vi "Master State Control.vi"(2 "Elevator_State":string) -> (0 "Elevator_State_Out":string, 1 "Target_Vacuum_Pump_Power":dbl)   [LabVIEW 2018]
uses:
  RefNumsDriverStation.vi
  Sensor Readings.vi
  Robot States.vi
panel:
  out "Target_Elevator_Position":dbl
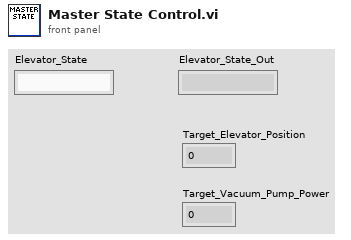
[diagram p1: front panel]
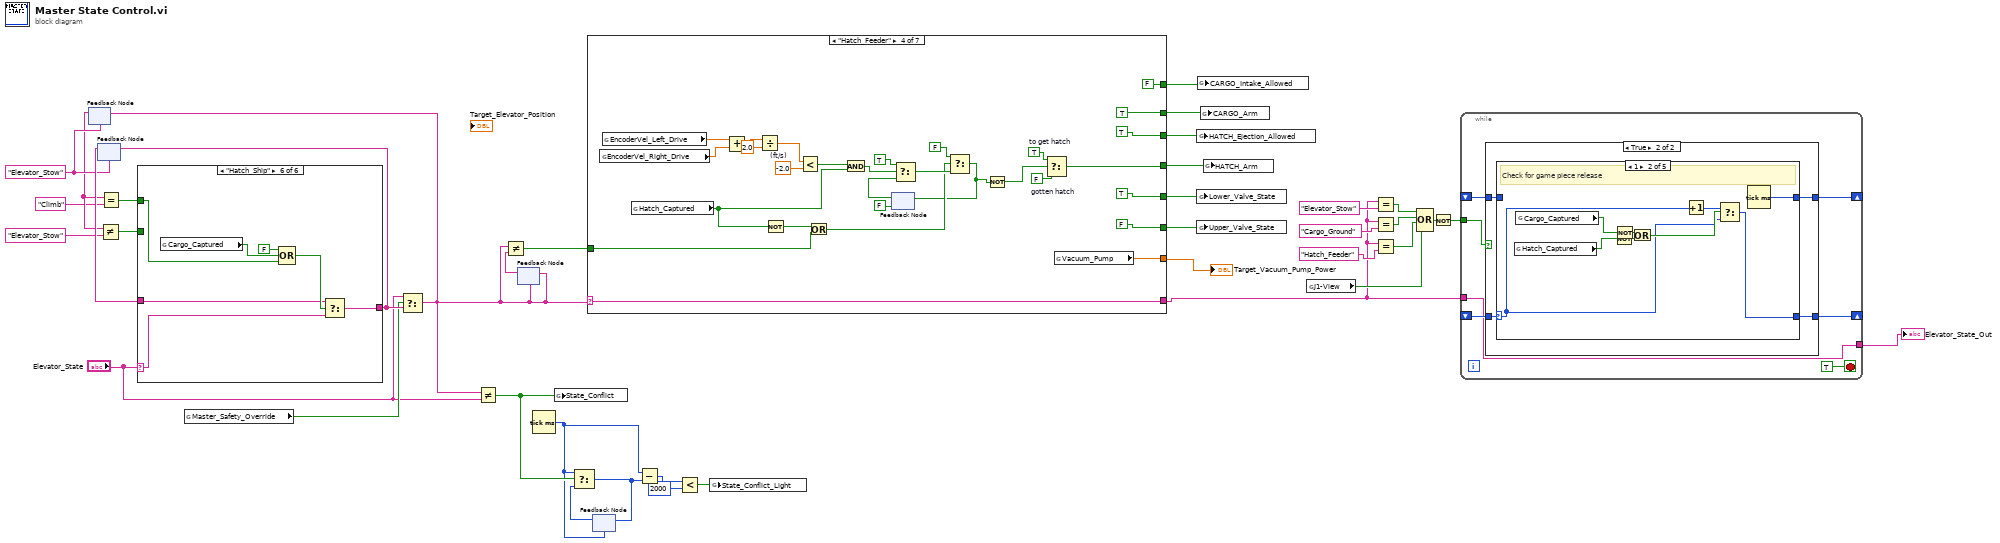
[diagram p0: block diagram]
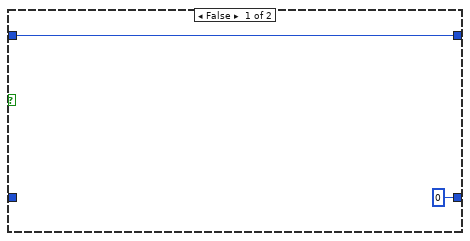
[diagram p2: hidden frame]
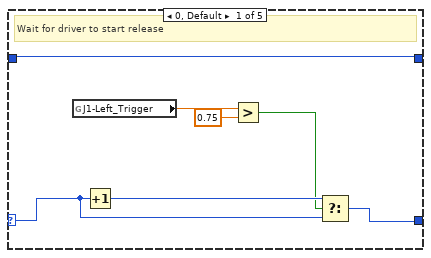
[diagram p3: hidden frame]
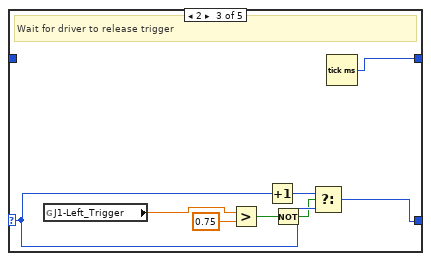
[diagram p4: hidden frame]
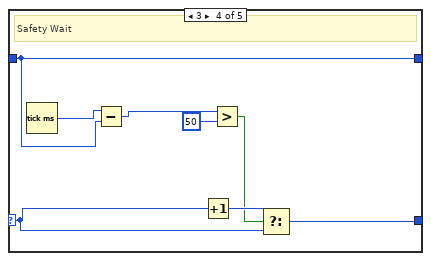
[diagram p5: hidden frame]
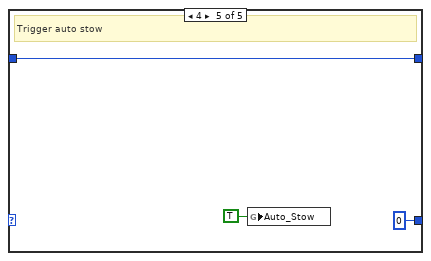
[diagram p6: hidden frame]
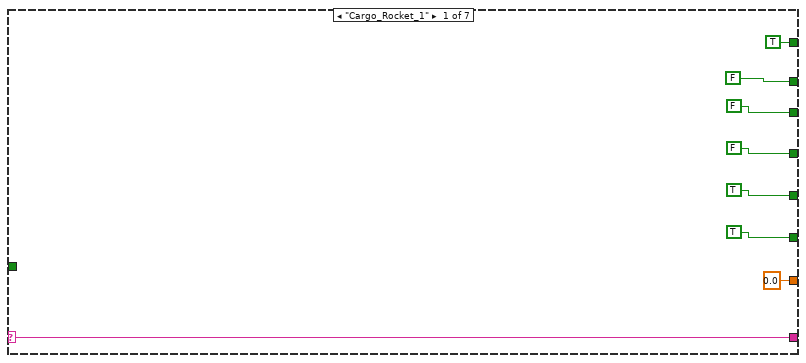
[diagram p7: hidden frame]
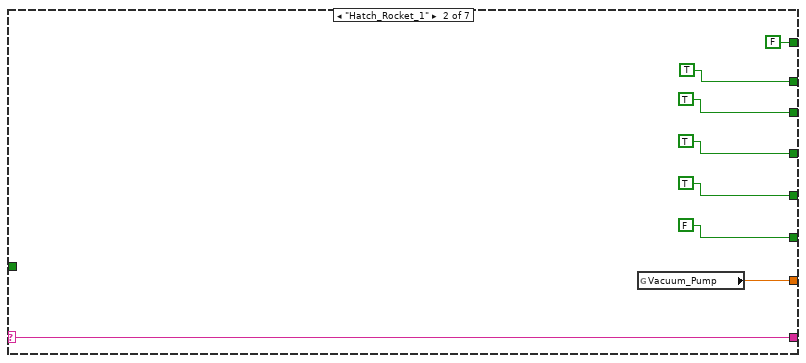
[diagram p8: hidden frame]
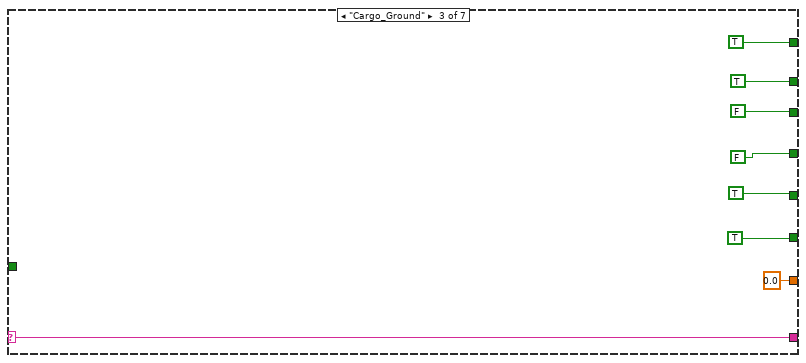
[diagram p9: hidden frame]
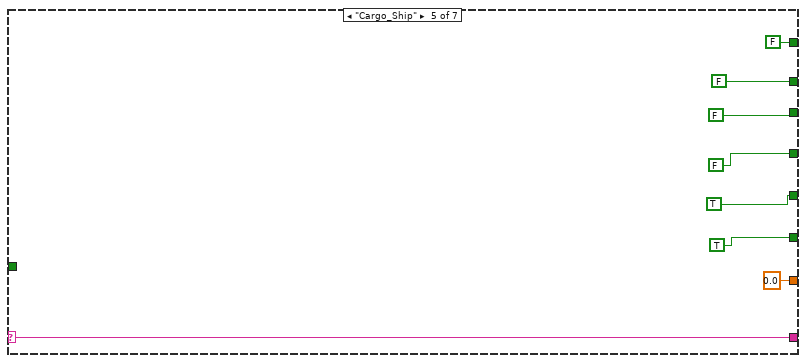
[diagram p10: hidden frame]
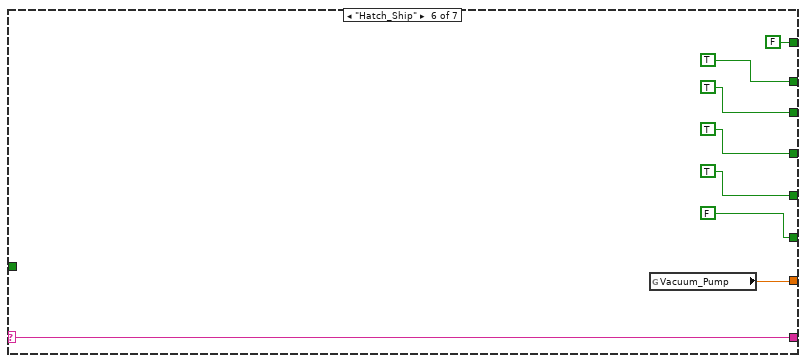
[diagram p11: hidden frame]
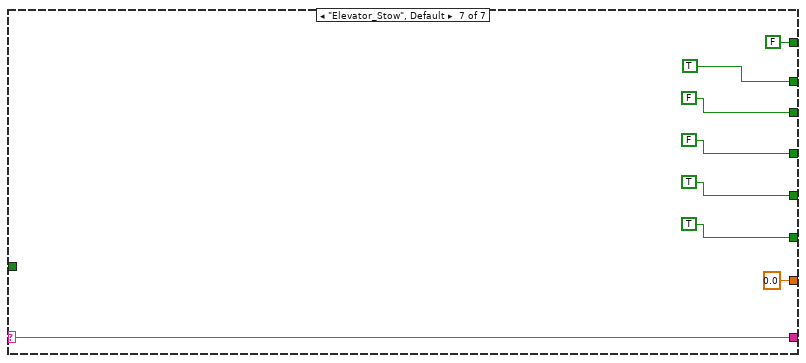
[diagram p12: hidden frame]
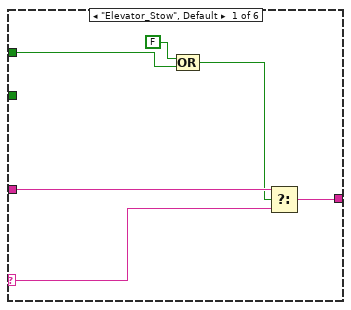
[diagram p13: hidden frame]
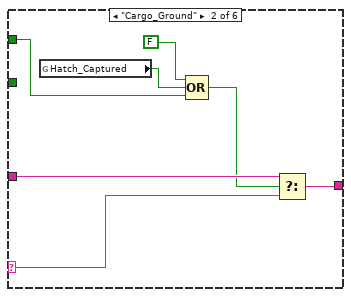
[diagram p14: hidden frame]
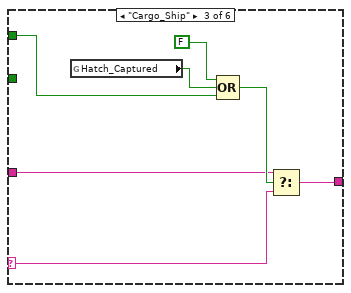
[diagram p15: hidden frame]
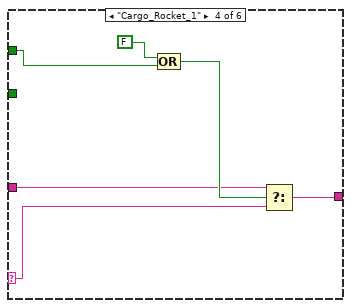
[diagram p16: hidden frame]
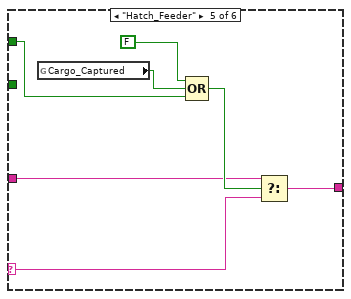
[diagram p17: hidden frame]
diagram:
  w36 = "Elevator_Stow" ("Elevator_State")
  n1 = feedback #1(w36) -> (w34:string)
  n2 = feedback #2(w36) -> (w38:string)
  n3 = Not Equal?(x=w34, y="Elevator_Stow") -> (x != y?=w32:bool)
  n4 = Equal?(x=w34, y="Climb") -> (x = y?=w31:bool)
  n5 = case shown="\"Hatch_Ship\"" "Elevator_State" {
    selector: "Elevator_State" -> [w39 w47 w54 w60 w66 w73]
    tunnel: [w44 w48 w55 w59 w65 w75] -> w37
    tunnel: w38 -> [w43 w46 w52 w61 w67 w72]
    tunnel: w32 -> [_ _ _ _ _ _]
    tunnel: w31 -> [w42 w51 w56 w64 w71 w78]
    frame "Elevator_Stow", Default {
      n6 = Compound Arithmetic op=OR(FALSE ("value"), w42) -> (w40:bool)
      n7 = Select(t=w43, s=w40, f=w39) -> (s? t:f=w44:string)
    }
    frame "Cargo_Ground" {
      n8 = global read "Sensor Readings.vi" "Hatch_Captured"() -> (w50:bool)
      n9 = Compound Arithmetic op=OR(FALSE ("value"), w50, w51) -> (w45:bool)
      n10 = Select(t=w46, s=w45, f=w47) -> (s? t:f=w48:string)
    }
    frame "Cargo_Ship" {
      n11 = global read "Sensor Readings.vi" "Hatch_Captured"() -> (w58:bool)
      n12 = Compound Arithmetic op=OR(FALSE ("value"), w58, w56) -> (w53:bool)
      n13 = Select(t=w52, s=w53, f=w54) -> (s? t:f=w55:string)
    }
    frame "Cargo_Rocket_1" {
      n14 = Compound Arithmetic op=OR(FALSE ("value"), w64) -> (w62:bool)
      n15 = Select(t=w61, s=w62, f=w60) -> (s? t:f=w59:string)
    }
    frame "Hatch_Feeder" {
      n16 = global read "Sensor Readings.vi" "Cargo_Captured"() -> (w70:bool)
      n17 = Compound Arithmetic op=OR(FALSE ("value"), w70, w71) -> (w68:bool)
      n18 = Select(t=w67, s=w68, f=w66) -> (s? t:f=w65:string)
    }
    frame "Hatch_Ship" {
      n19 = global read "Sensor Readings.vi" "Cargo_Captured"() -> (w77:bool)
      n20 = Compound Arithmetic op=OR(FALSE ("value"), w77, w78) -> (w74:bool)
      n21 = Select(t=w72, s=w74, f=w73) -> (s? t:f=w75:string)
    }
  }
  n22 = feedback-in #2(w37) -> ()
  n23 = global read "RefNumsDriverStation.vi" "Master_Safety_Override"() -> (w12:bool)
  n24 = Select(t="Elevator_State", s=w12, f=w37) -> (s? t:f=w1:string)
  n25 = feedback-in #1(w1) -> ()
  n26 = Not Equal?(x=w1, y="Elevator_State") -> (x != y?=w10:bool)
  n27 = feedback-in #3(w1) -> ()
  n28 = feedback #3(w1) -> (w3:string)
  n29 = Not Equal?(x=w1, y=w3) -> (x != y?=w2:bool)
  n30 = Tick Count (ms)() -> (millisecond timer value=w5:u32)
  n31 = global write "Robot States.vi" "State_Conflict"(w10) -> ()
  n32 = case shown="\"Hatch_Feeder\"" w1 {
    selector: w1 -> [w79 w94 w102 w131 w139 w147 w155]
    tunnel: [w79 w94 w102 w131 w139 w147 w155] -> w13
    tunnel: [0.0 ("Vacuum_Pump") w93 0.0 ("Vacuum_Pump") w130 0.0 ("Vacuum_Pump") w146 0.0 ("Vacuum_Pump")] -> w30
    tunnel: [FALSE TRUE FALSE TRUE FALSE TRUE FALSE] -> w29
    tunnel: [FALSE TRUE FALSE w103 FALSE TRUE FALSE] -> w28
    tunnel: [TRUE TRUE TRUE TRUE TRUE TRUE TRUE] -> w27
    tunnel: [TRUE FALSE TRUE FALSE TRUE FALSE TRUE] -> w26
    tunnel: [FALSE ("CARGO_Arm") TRUE ("CARGO_Arm") TRUE ("CARGO_Arm") TRUE ("CARGO_Arm") FALSE ("CARGO_Arm") TRUE ("CARGO_Arm") TRUE ("CARGO_Arm")] -> w25
    tunnel: [TRUE ("CARGO_Intake_Allowed") FALSE ("CARGO_Intake_Allowed") TRUE ("CARGO_Intake_Allowed") FALSE ("CARGO_Intake_Allowed") FALSE ("CARGO_Intake_Allowed") FALSE ("CARGO_Intake_Allowed") FALSE ("CARGO_Intake_Allowed")] -> w24
    tunnel: w2 -> [_ _ _ w111 _ _ _]
    frame "Cargo_Rocket_1" {
    }
    frame "Hatch_Rocket_1" {
      n33 = global read "RefNumsDriverStation.vi" "Vacuum_Pump"() -> (w93:dbl)
    }
    frame "Cargo_Ground" {
    }
    frame "Hatch_Feeder" {
      w105 = TRUE  # to get hatch
      w104 = FALSE  # gotten hatch
      w119 = -2.0  # (ft/s)
      n34 = global read "Sensor Readings.vi" "EncoderVel_Right_Drive"() -> (w123:dbl)
      n35 = global read "Sensor Readings.vi" "EncoderVel_Left_Drive"() -> (w124:dbl)
      n36 = global read "Sensor Readings.vi" "Hatch_Captured"() -> (w109:bool)
      n37 = Add(x=w124, y=w123) -> (x+y=w122:dbl)
      n38 = Divide(x=w122, y=2.0) -> (x/y=w120:dbl)
      n39 = Not(x=w109) -> (.not. x?=w110:bool)
      n40 = Less?(x=w120, y=w119) -> (x < y?=w118:bool)
      n41 = Or(x=w110, y=w111) -> (x .or. y?=w108:bool)
      n42 = And(x=w118, y=w109) -> (x .and. y?=w117:bool)
      n43 = feedback #4(FALSE) -> (w116:bool)
      n44 = Select(t=TRUE, s=w117, f=w116) -> (s? t:f=w114:bool)
      n45 = Select(t=FALSE, s=w108, f=w114) -> (s? t:f=w107:bool)
      n46 = feedback-in #4(w107) -> ()
      n47 = Not(x=w107) -> (.not. x?=w106:bool)
      n48 = Select(t=w105, s=w106, f=w104) -> (s? t:f=w103:bool)
      n49 = global read "RefNumsDriverStation.vi" "Vacuum_Pump"() -> (w130:dbl)
    }
    frame "Cargo_Ship" {
    }
    frame "Hatch_Ship" {
      n50 = global read "RefNumsDriverStation.vi" "Vacuum_Pump"() -> (w146:dbl)
    }
    frame "Elevator_Stow", Default {
    }
  }
  "Target_Vacuum_Pump_Power" <- w30
  n51 = feedback #5(w5) -> (w6:u32)
  n52 = Select(t=w5, s=w10, f=w6) -> (s? t:f=w7:u32)
  n53 = feedback-in #5(w7) -> ()
  n54 = Subtract(x=w5, y=w7) -> (x-y=w9:u32)
  n55 = Less?(x=w9, y=u32 2000) -> (x < y?=w4:bool)
  n56 = global write "Robot States.vi" "State_Conflict_Light"(w4) -> ()
  n57 = global write "Robot States.vi" "HATCH_Ejection_Allowed"(w29) -> ()
  n58 = global write "Robot States.vi" "Lower_Valve_State"(w27) -> ()
  n59 = global write "Robot States.vi" "Upper_Valve_State"(w26) -> ()
  n60 = global write "Robot States.vi" "CARGO_Intake_Allowed"(w24) -> ()
  n61 = global write "Robot States.vi" "CARGO_Arm"(w25) -> ()
  n62 = global write "Robot States.vi" "HATCH_Arm"(w28) -> ()
  n63 = global read "RefNumsDriverStation.vi" "J1-View"() -> (w17:bool)
  n64 = Equal?(x=w13, y="Elevator_Stow") -> (x = y?=w20:bool)
  n65 = Equal?(x=w13, y="Cargo_Ground") -> (x = y?=w19:bool)
  n66 = Equal?(x=w13, y="Hatch_Feeder") -> (x = y?=w18:bool)
  n67 = Compound Arithmetic op=OR(w20, w19, w18, w17) -> (w16:bool)
  n68 = Not(x=w16) -> (.not. x?=w15:bool)
  n69 = while {
    tunnel: w15 -> [w162]
    shift-right: [w160] -> _
    shift-left: _ -> [w161]
    shift-right: [w159] -> _
    shift-left: _ -> [w158]
    tunnel: [w156] -> w14
    tunnel: w13 -> [w156]
    stop <- TRUE stop-if-true
    n70 = case shown="True" w162 {
      tunnel: w161 -> [_ w168]
      tunnel: [0 w167] -> w160
      tunnel: [w164 w166] -> w159
      tunnel: w158 -> [w164 w165]
      frame False {
      }
      frame True {
        n71 = case shown="1" w168 {
          selector: w168 -> [w174 w178 w190 w196 _]
          tunnel: [w173 w176 w187 w194 0] -> w167
          tunnel: [w172 w177 w188 w193 w203] -> w166
          tunnel: w165 -> [w172 _ _ w193 w203]
          frame 0, Default {
            # "Wait for driver to start release"
            n72 = global read "RefNumsDriverStation.vi" "J1-Left_Trigger"() -> (w171:dbl)
            n73 = Increment(x=w174) -> (x+1=w175:i32)
            n74 = Greater?(x=w171, y=0.75) -> (0:w169:bool)
            n75 = Select(t=w175, s=w169, f=w174) -> (s? t:f=w173:i32)
          }
          frame 1 {
            # "Check for game piece release"
            n76 = global read "Sensor Readings.vi" "Hatch_Captured"() -> (w183:bool)
            n77 = global read "Sensor Readings.vi" "Cargo_Captured"() -> (w184:bool)
            n78 = Not(x=w183) -> (.not. x?=w181:bool)
            n79 = Not(x=w184) -> (.not. x?=w182:bool)
            n80 = Or(x=w182, y=w181) -> (x .or. y?=w179:bool)
            n81 = Increment(x=w178) -> (x+1=w180:i32)
            n82 = Select(t=w180, s=w179, f=w178) -> (s? t:f=w176:i32)
            n83 = Tick Count (ms)() -> (millisecond timer value=w177:u32)
          }
          frame 2 {
            # "Wait for driver to release trigger"
            n84 = global read "RefNumsDriverStation.vi" "J1-Left_Trigger"() -> (w186:dbl)
            n85 = Greater?(x=w186, y=0.75) -> (0:w189:bool)
            n86 = Increment(x=w190) -> (x+1=w191:i32)
            n87 = Not(x=w189) -> (.not. x?=w185:bool)
            n88 = Select(t=w191, s=w185, f=w190) -> (s? t:f=w187:i32)
            n89 = Tick Count (ms)() -> (millisecond timer value=w188:u32)
          }
          frame 3 {
            # "Safety Wait"
            n90 = Tick Count (ms)() -> (millisecond timer value=w200:u32)
            n91 = Subtract(x=w200, y=w193) -> (x-y=w199:u32)
            n92 = Increment(x=w196) -> (x+1=w197:i32)
            n93 = Greater?(x=w199, y=u32 50) -> (0:w195:bool)
            n94 = Select(t=w197, s=w195, f=w196) -> (s? t:f=w194:i32)
          }
          frame 4 {
            # "Trigger auto stow"
            n95 = global write "Robot States.vi" "Auto_Stow"(TRUE ("Auto_Stow")) -> ()
          }
        }
      }
    }
  }
  "Elevator_State_Out" <- w14
